vi "Partial Fraction Expansion.vi"(8 "option":u16(ring) items=["Cancel Co-factors", "Reserve Co-factors"], 9 "tolerance":dbl=1e-05, 10 "Denominator":cdb[](array[numeric]) format="%#.6g", 11 "Numerator":cdb[](array[numeric]) format="%#.6g") -> (0 "error":i32, 1 "Residues":cdb[][](array[numeric]) format="%#.6g", 2 "Poles":cdb[](array[numeric]) format="%#.6g", 3 "Polynomial":cdb[](array[numeric]) format="%#.6g", 5 "Multiplicity":i32[](array[numeric]))   [LabVIEW 2014, in "NI_AALPro.lvlib"]
doc: "Calculates the partial fraction expansion of a polynomial using the Heaviside cover-up method."
uses:
  NI_AALPro.lvlib
  Remove Zero Coefficients (CDB).vi
  Divide Polynomials (CDB).vi
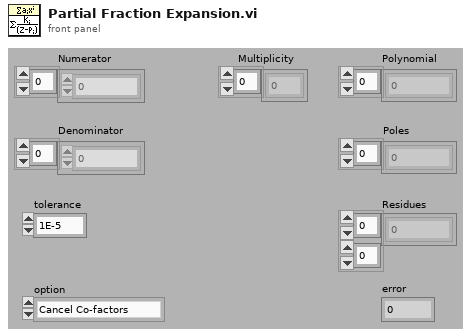
[diagram p1: front panel]
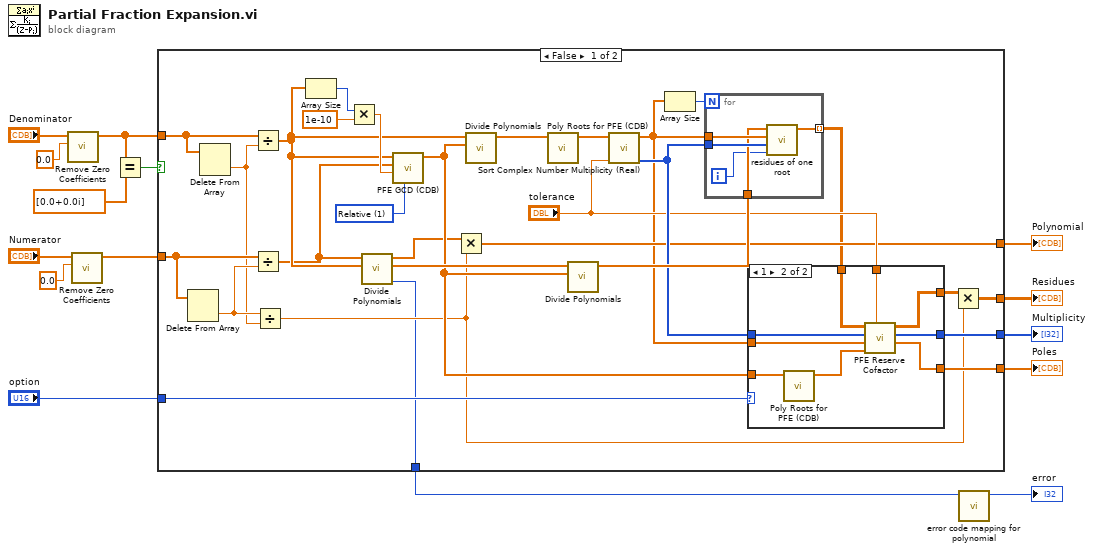
[diagram p0: block diagram]
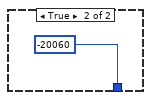
[diagram p3: hidden frame]
diagram:
  n1 = call-poly "Remove Zero Coefficients.vi"("threshold"=0.0, "P(x) In"="Denominator") -> ("P(x) Out"=w2:cdb[])  [unwired: 7 in, 2 out]
  n2 = call-poly "Remove Zero Coefficients.vi"("threshold"=0.0, "P(x) In"="Numerator") -> ("P(x) Out"=w8:cdb[])  [unwired: 7 in, 2 out]
  n3 = Equal?(x=w2, y=cdb[] [0.0+0.0i] ("P(x) Out")) -> (x = y?=w3:bool)
  n4 = case shown="False" w3 {
    tunnel: "option" -> [w40 _]
    tunnel: [w38 _] -> w10
    tunnel: [w37 _] -> w9
    tunnel: w2 -> [w31 _]
    tunnel: w8 -> [w29 _]
    tunnel: [w25 _] -> w7
    tunnel: [w19 _] -> w6
    tunnel: [w18 -20060] -> w4
    frame False {
      w32 = u16 1 items=["Absolute", "Relative"] ("tolerance type")
      n5 = Delete From Array(array=w29) -> (deleted portion=w27:cdb)  [unwired: 2 in, 1 out]
      n6 = Delete From Array(array=w31) -> (deleted portion=w26:cdb)  [unwired: 2 in, 1 out]
      n7 = Divide(x=w31, y=w26) -> (x/y=w30:cdb[])
      n8 = Divide(x=w29, y=w27) -> (x/y=w28:cdb[])
      n9 = Divide(x=w27, y=w26) -> (x/y=w20:cdb)
      n10 = Array Size(array=w30) -> (size(s)=w43:i32)
      n11 = Multiply(x=w43, y=1e-10 ("eps for GCD")) -> (x*y=w34:dbl)
      n12 = call-poly "Divide Polynomials.vi"("Q(x)"=w30, "P(x)"=w28) -> ("error"=w18:i32, "Remainder"=w42:cdb[], "P(x)/Q(x)"=w24:cdb[])  [unwired: 7 in]
      n13 = call "PFE GCD (CDB).vi"("tolerance type"=w32, "tolerance"=w34, "Q(x)"=w28, "P(x)"=w30) -> ("Greatest Common Divisor"=w33:cdb[])  [unwired: 6 in, 1 out]
      n14 = Multiply(x=w24, y=w20) -> (x*y=w25:cdb[])
      n15 = call-poly "Divide Polynomials.vi"("Q(x)"=w33, "P(x)"=w30) -> ("P(x)/Q(x)"=w23:cdb[])  [unwired: 7 in, 2 out]
      n16 = call "Poly Roots for PFE (CDB).vi"("P(x)"=w23) -> ("Roots"=w35:cdb[])  [unwired: 10 in]
      n17 = call-poly "Divide Polynomials.vi"("Q(x)"=w33, "P(x)"=w42) -> ("P(x)/Q(x)"=w41:cdb[])  [unwired: 7 in, 2 out]
      n18 = call "Sort Complex Number Multiplicity (Real).vi"("tolerance"="tolerance", "Complex numbers"=w35) -> ("Multiplicity"=w39:i32[], "Sorted unique complex numbers"=w16:cdb[])  [unwired: 8 in]
      n19 = Array Size(array=w16) -> (size(s)=w17:i32)
      n20 = for {
        N: w17 -> [_]
        tunnel: w39 -> [w59]
        tunnel: w16 -> [w60]
        tunnel: w41 -> [w58]
        tunnel: [w61] -> w22 mode=indexing
        i -> [w57]
        n21 = call "residues of one root.vi"("index of root"=w57, "multiplicity of roots"=w59, "roots"=w60, "Rest"=w58) -> ("Residues of root"=w61:cdb[])  [unwired: 7 in]
      }
      n22 = case shown="1" w40 {
        tunnel: w39 -> [w47 w55]
        tunnel: w16 -> [w46 w56]
        tunnel: [w46 w50] -> w38
        tunnel: [w47 w51] -> w37
        tunnel: w33 -> [_ w49]
        tunnel: w22 -> [w45 w54]
        tunnel: [w45 w52] -> w21
        tunnel: "tolerance" -> [_ w53]
        frame 0, Default {
        }
        frame 1 {
          n23 = call "Poly Roots for PFE (CDB).vi"("P(x)"=w49) -> ("Roots"=w48:cdb[])  [unwired: 10 in]
          n24 = call "PFE Reserve Cofactor.vi"("tolerance"=w53, "Co-factor Poles"=w48, "Poles In"=w56, "Multiplicity In"=w55, "Residues In"=w54) -> ("Poles Out"=w50:cdb[], "Multiplicity Out"=w51:i32[], "Residues Out"=w52:cdb[][])  [unwired: 4 in]
        }
      }
      n25 = Multiply(x=w21, y=w20) -> (x*y=w19:cdb[][])
    }
    frame True {
    }
  }
  "Poles" <- w10
  "Multiplicity" <- w9
  "Residues" <- w6
  "Polynomial" <- w7
  n26 = call "error code mapping for polynomial.vi"("error in"=w4) -> ("error out"=→"error":i32)  [unwired: 10 in]
